vi "SNA Convert Parameter to String.vi"(10 "Parameter":T1 {"Stimulus Port" min=1 step=1; "Response Port" min=1 step=1}) -> (2 "Parameter String":string)   [LabVIEW 2011]
uses:
  tests/S Parameter/TypeDefs/SP Parameter.ctl
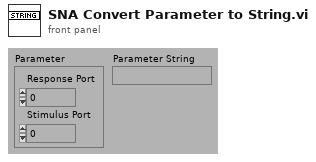
[diagram p1: front panel]
types:
  T1 = typedef "SP Parameter.ctl" = cluster{"Stimulus Port":i8, "Response Port":i8}
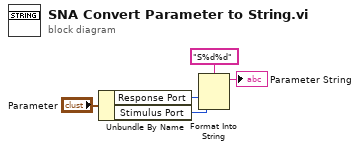
[diagram p0: block diagram]
diagram:
  n1 = Unbundle By Name("Parameter") -> ("Response Port"=w4:i8, "Stimulus Port"=w5:i8)
  n2 = Format Into String(format string="S%d%d", w4, w5) -> (resulting string=→"Parameter String":string)  [unwired: 2 in, 1 out]
